vi "Open Builder.vi"() -> (0 "error out":errorcluster, 3 "Builder out":refnum<class "Builder.lvclass">)   [LabVIEW 2021, in "App-Builder Library.lvlib" / "Builder.lvclass"]
uses:
  Builder.lvclass
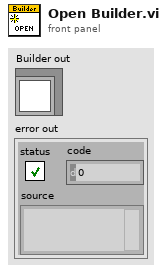
[diagram p1: front panel]
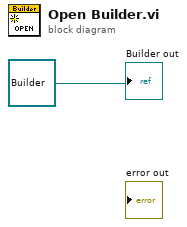
[diagram p0: block diagram]
diagram:
  "Builder out" <- refnum<class "Builder.lvclass"> refnum ("Builder in")
